vi "DS1104PlusDemo - 副本.vi"() -> ()   [LabVIEW 2018]
panel:
  out "错误输出":errorcluster
  in  "接口类型":u16(ring)=1 items=[""=0, "GPIB"=1, "VXI"=2, "GPIB-VXI"=3, "Serial"=4, "PXI"=5, "TCPIP"=6, "USB"=7, "FireWire"=9]
  in  "SINGLE Trigger":bool
  in  "RUN/STOP":bool
  in  "AUTO Set":bool
  in  "CLEAR Display":bool
  in  "Vertical Coupling":u16(ring) items=["AC", "DC", "Ground"]
  in  "Probe Attenuation":u16(ring) items=["1x"=1, "10x"=10]
  out "Single":bool caption="SINGLE"
  out "Normal":bool caption="NORMAL"
  out "Auto":bool caption="AUTO"
  in  "Trigger MODE":string(combo)
  in  "FORCE Trigger":bool
  in  "Trigger MENU":bool
  in  "Trigger LEVEL":dbl(ring)
  in  "Horizontal POSITION":ext format="%#_9g"
  in  "Horizontal MENU":bool
  in  "Horizaontal SCALE":ext(ring)=1e-09 items=["1u", "2u", "5u", "10u", "20u", "50u", "100u", "200u", "500u", "1m", "2m", "5m", "10m", "20m", "50m", "100m", "200m", "500m", "1", "2", "5", "10", "20", "50", "100", "200", "500", "1000"]
  in  "REF":bool
  in  "MATH":bool
  in  "Vertical SCALE":dbl(ring) items=["500u"=0.0005, "1m"=0.001, "2m"=0.002, "5m"=0.005, "10m"=0.01, "20m"=0.02, "50m"=0.05, "100m"=0.1, "200m"=0.2, "500m"=0.5, "1"=1.0, "2"=2.0, "5"=5.0, "10"=10.0, "20"=20.0, "50"=50.0, "100"=100.0]
  in  "Vertical POSITION":dbl min=-100.0 max=100.0 step=0.1 format="%#_4g"
  in  "CH4":bool
  in  "CH3":bool
  in  "CH2":bool
  in  "CH1":bool
  out "波形图":waveform(dbl)(graph)
  in  "VISA资源名称":refnum<visa-resource-name>
  # "VERTICAL"
  # "HORIZONTAL"
  # "TRIGGER"
  # "POSITION"
  # "POSITION"
  # "s"
  # "V"
  # "SCALE"
  # "SCALE"
  # "s/div"
  # "V/div"
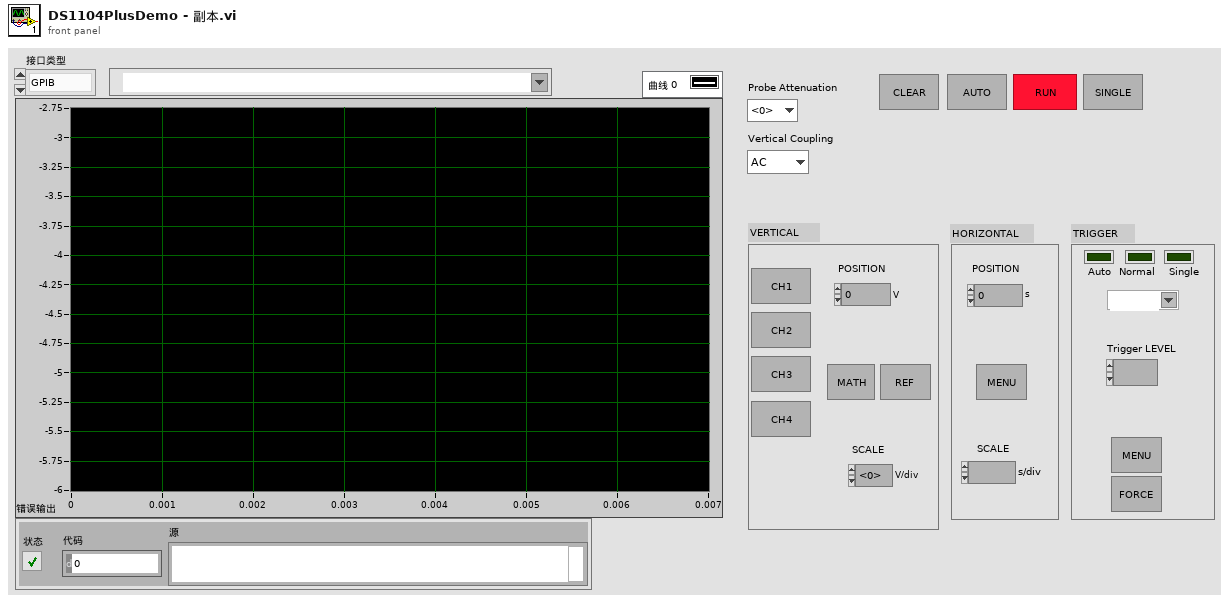
[diagram p1: front panel]
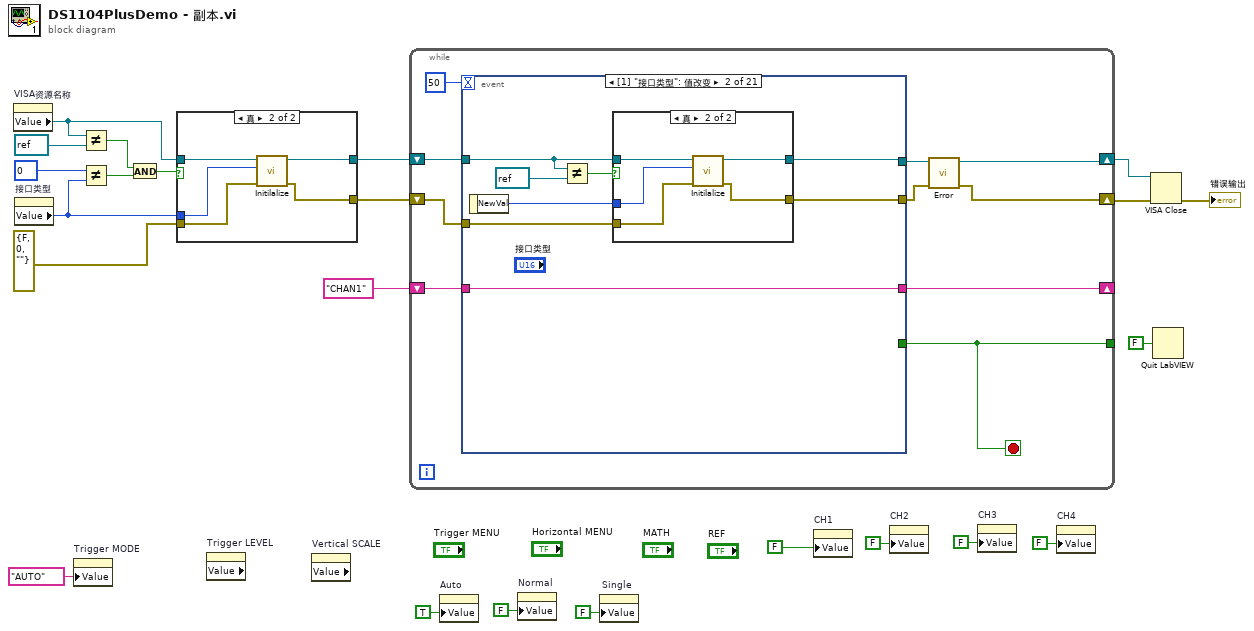
[diagram p0: block diagram]
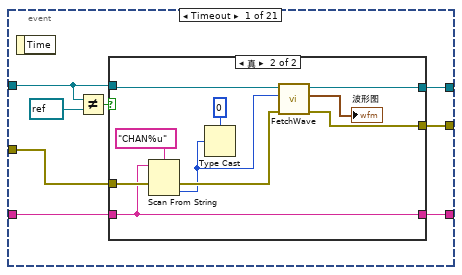
[diagram p3: hidden frame]
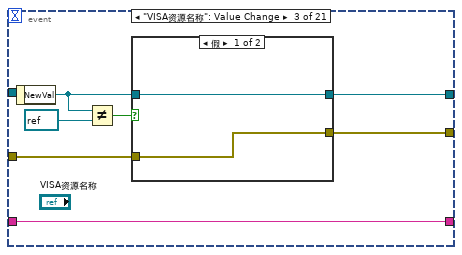
[diagram p6: hidden frame]
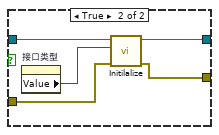
[diagram p7: hidden frame]
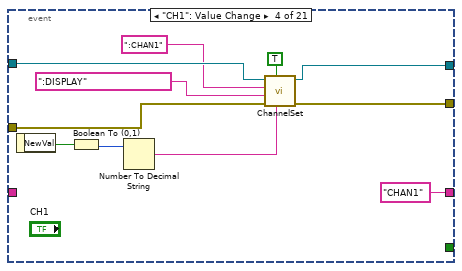
[diagram p8: hidden frame]
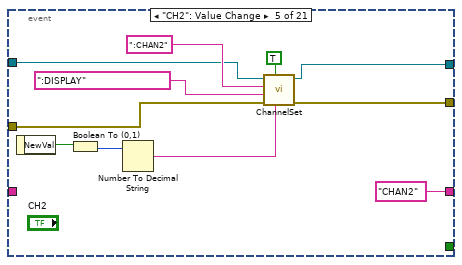
[diagram p9: hidden frame]
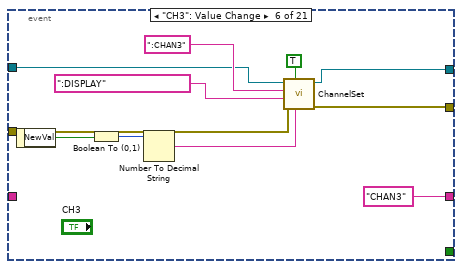
[diagram p10: hidden frame]
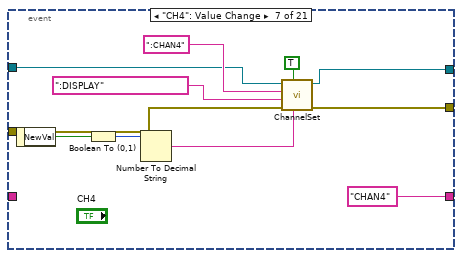
[diagram p11: hidden frame]
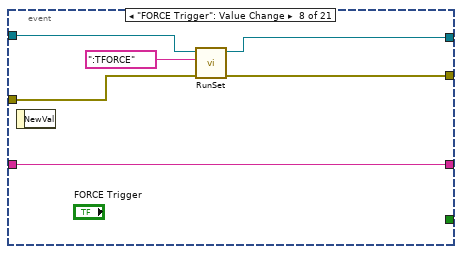
[diagram p12: hidden frame]
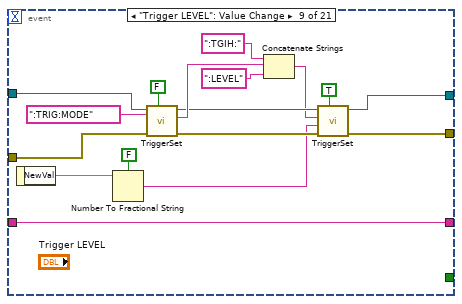
[diagram p13: hidden frame]
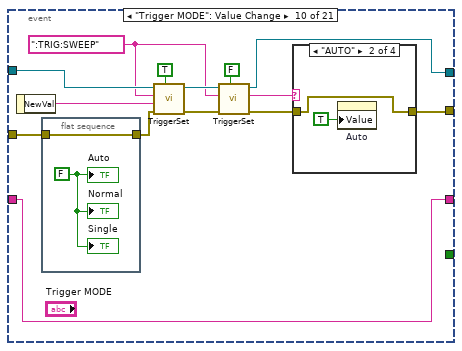
[diagram p14: hidden frame]
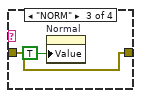
[diagram p16: hidden frame]
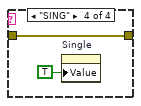
[diagram p17: hidden frame]
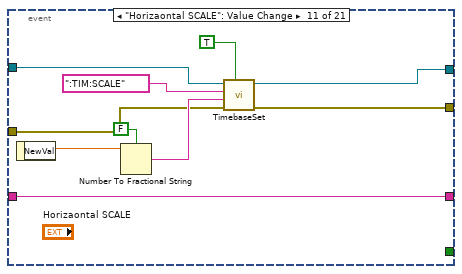
[diagram p18: hidden frame]
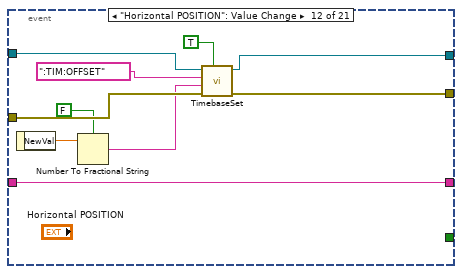
[diagram p19: hidden frame]
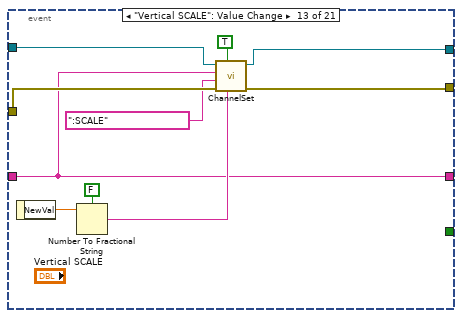
[diagram p20: hidden frame]
diagram:
  w12 = u16 0 items=[""=0, "GPIB"=1, "VXI"=2, "GPIB-VXI"=3, "Serial"=4, "PXI"=5, "TCPIP"=6, "USB"=7, "FireWire"=9] ("接口类型")
  n1 = property on="VISA资源名称" class="VISAName"() -> ("Value"=w13:refnum<visa-resource-name>)  [unwired: 2 in, 2 out]
  n2 = property on="接口类型" class="Ring (严格)"() -> ("Value"=w11:u16)  [unwired: 2 in, 2 out]
  n3 = property on="Trigger MODE" class="CmbBox"("Value"="AUTO" ("Trigger MODE")) -> ()  [unwired: 2 in, 2 out]
  n4 = Not Equal?(x=w13, y=refnum<visa-resource-name> refnum ("VISA引用句柄输出")) -> (x != y?=w16:bool)
  n5 = Not Equal?(x=w12, y=w11) -> (x != y?=w15:bool)
  n6 = And(x=w16, y=w15) -> (x .and. y?=w17:bool)
  n7 = case shown="真" w17 {
    tunnel: w13 -> [w25 w30]
    tunnel: errorcluster {"status"=FALSE, "code"=0, "source"=""} ("错误常量") -> [w24 w29]
    tunnel: w11 -> [_ w28]
    tunnel: [w24 w27] -> w9
    tunnel: [w25 w26] -> w10
    frame False {
    }
    frame True {
      n8 = call "Initilalize.vi"("错误输入（无错误）"=w29, "接口类型"=w28, "VISA资源名称"=w30) -> ("错误输出"=w27:errorcluster, "VISA资源名称输出"=w26:refnum<visa-resource-name>)  [unwired: 7 in]
    }
  }
  n9 = property on="Trigger LEVEL" class="Ring (严格)" props=["Value"]() -> ()  [unwired: 2 in, 3 out]
  n10 = property on="Vertical SCALE" class="Ring (严格)" props=["Value"]() -> ()  [unwired: 2 in, 3 out]
  n11 = while {
    shift-right: [w32] -> w8
    shift-left: w10 -> [w39]
    shift-right: [w33] -> w7
    shift-left: w9 -> [w38]
    shift-right: [w36] -> _
    shift-left: "CHAN1" ("通道选择") -> [w37]
    tunnel: [w31] -> _
    stop <- w31 stop-if-true
    n12 = event shown="[1] \"接口类型\": 值改变" {
      selector: _ -> [_ _ _ _ _ _ _ _ _ _ _ _ _ _ _ _ _ _ _ _ _]
      dyn-events: _ -> [_ _ _ _ _ _ _ _ _ _ _ _ _ _ _ _ _ _ _ _ _]
      timeout: 50 -> [_ _ _ _ _ _ _ _ _ _ _ _ _ _ _ _ _ _ _ _ _]
      tunnel: w39 -> [w42 w66 _ w101 w106 w119 w130 w138 w156 w171 w190 w199 w210 w218 w230 w236 w243 w249 w259 w264 w270]
      tunnel: w38 -> [w47 w65 w79 w100 w105 w118 w129 w139 w155 w159 w184 w200 w209 w217 w228 w239 w242 w250 w258 w265 w269]
      tunnel: [w46 w62 w78 w93 w104 w117 w128 w135 w141 w160 w183 w194 w204 w213 w227 w237 w241 w248 w257 w262 w267] -> w35
      tunnel: [w45 w63 w77 w92 w103 w116 w127 w137 w142 w161 w182 w193 w202 w212 w226 w238 w240 w247 w256 w261 w268] -> w34
      tunnel: w37 -> [w48 w69 w83 _ _ _ _ w140 w157 w170 w181 w192 w205 w211 w224 w235 w245 w251 w260 w266 w272]
      tunnel: [w41 w69 w83 "CHAN1" ("通道选择") "CHAN2" ("通道选择") "CHAN3" ("通道选择") "CHAN4" ("通道选择") w140 w157 w170 w181 w192 w205 w211 w224 w235 w245 w251 w260 w266 w271] -> w36
      tunnel: [_ _ _ _ _ _ _ _ _ _ _ _ _ _ _ _ _ _ _ _ w273] -> w31
      event Timeout {
        n13 = event-data() -> ()  [unwired: 1 in, 1 out]
        n14 = Not Equal?(x=w42, y=refnum<visa-resource-name> refnum) -> (x != y?=w44:bool)
        n15 = case shown="真" w44 {
          tunnel: w48 -> [w49 w54]
          tunnel: w47 -> [w50 w60]
          tunnel: [w51 w58] -> w46
          tunnel: [w50 w57] -> w45
          tunnel: w42 -> [w51 w55]
          tunnel: [w49 w54] -> w41
          frame False {
          }
          frame True {
            n16 = Scan From String(format string="CHAN%u" ("格式字符串"), input string=w54, error in=w60) -> (error out=w59:errorcluster, output 1=w52:u32)  [unwired: 2 in, 2 out]
            n17 = Type Cast(type=u16 0, x=w52) -> ()  [unwired: 1 out]
            n18 = call "FetchWave.vi"("error in (no error)"=w59, "通道"=w52, "VISA资源名称"=w55) -> ("error out"=w57:errorcluster, "波形图"=→"波形图":waveform(dbl), "VISA资源名称 2"=w58:refnum<visa-resource-name>)  [unwired: 6 in]
          }
        }
      }
      event "接口类型": Value Change {
        n19 = event-data() -> ("NewVal"=w64:u16)  [unwired: 1 in]
        n20 = Not Equal?(x=w66, y=refnum<visa-resource-name> refnum ("VISA引用句柄输出")) -> (x != y?=w67:bool)
        n21 = case shown="真" w67 {
          tunnel: w66 -> [w71 w76]
          tunnel: w65 -> [w70 w75]
          tunnel: w64 -> [_ w74]
          tunnel: [w70 w73] -> w63
          tunnel: [w71 w72] -> w62
          frame False {
          }
          frame True {
            n22 = call "Initilalize.vi"("错误输入（无错误）"=w75, "接口类型"=w74, "VISA资源名称"=w76) -> ("错误输出"=w73:errorcluster, "VISA资源名称输出"=w72:refnum<visa-resource-name>)  [unwired: 7 in]
          }
        }
      }
      event "VISA资源名称": Value Change {
        n23 = event-data() -> ("NewVal"=w80:refnum<visa-resource-name>)  [unwired: 1 in]
        n24 = Not Equal?(x=w80, y=refnum<visa-resource-name> refnum ("VISA引用句柄输出")) -> (x != y?=w81:bool)
        n25 = case shown="假" w81 {
          tunnel: w80 -> [w85 w90]
          tunnel: w79 -> [w84 w88]
          tunnel: [w85 w87] -> w78
          tunnel: [w84 w86] -> w77
          frame False {
          }
          frame True {
            n26 = property on="接口类型" class="Ring (严格)"() -> ("Value"=w89:u16)  [unwired: 2 in, 2 out]
            n27 = call "Initilalize.vi"("错误输入（无错误）"=w88, "接口类型"=w89, "VISA资源名称"=w90) -> ("错误输出"=w86:errorcluster, "VISA资源名称输出"=w87:refnum<visa-resource-name>)  [unwired: 7 in]
          }
        }
      }
      event "CH1": Value Change {
        n28 = event-data() -> ("NewVal"=w96:bool)  [unwired: 1 in]
        n29 = Boolean To (0,1)(Boolean=w96) -> (0, 1=w95:i16)
        n30 = Number To Decimal String(number=w95) -> (decimal integer string=w94:string)  [unwired: 1 in]
        n31 = call "ChannelSet.vi"("设置参数"=w94, "参数查询(0)/设置(1)"=TRUE, "error in (no error)"=w100, "CHANNLE命令子系统"=":DISPLAY", "通道选择"=":CHAN1", "VISA资源名称"=w101) -> ("error out"=w92:errorcluster, "VISA资源名称 2"=w93:refnum<visa-resource-name>)  [unwired: 2 in, 2 out]
      }
      event "CH2": Value Change {
        n32 = event-data() -> ("NewVal"=w102:bool)  [unwired: 1 in]
        n33 = Boolean To (0,1)(Boolean=w102) -> (0, 1=w110:i16)
        n34 = Number To Decimal String(number=w110) -> (decimal integer string=w109:string)  [unwired: 1 in]
        n35 = call "ChannelSet.vi"("设置参数"=w109, "参数查询(0)/设置(1)"=TRUE, "error in (no error)"=w105, "CHANNLE命令子系统"=":DISPLAY", "通道选择"=":CHAN2", "VISA资源名称"=w106) -> ("error out"=w103:errorcluster, "VISA资源名称 2"=w104:refnum<visa-resource-name>)  [unwired: 2 in, 2 out]
      }
      event "CH3": Value Change {
        n36 = event-data() -> ("NewVal"=w114:bool)  [unwired: 1 in]
        n37 = Boolean To (0,1)(Boolean=w114) -> (0, 1=w113:i16)
        n38 = Number To Decimal String(number=w113) -> (decimal integer string=w121:string)  [unwired: 1 in]
        n39 = call "ChannelSet.vi"("设置参数"=w121, "参数查询(0)/设置(1)"=TRUE, "error in (no error)"=w118, "CHANNLE命令子系统"=":DISPLAY", "通道选择"=":CHAN3", "VISA资源名称"=w119) -> ("error out"=w116:errorcluster, "VISA资源名称 2"=w117:refnum<visa-resource-name>)  [unwired: 2 in, 2 out]
      }
      event "CH4": Value Change {
        n40 = event-data() -> ("NewVal"=w125:bool)  [unwired: 1 in]
        n41 = Boolean To (0,1)(Boolean=w125) -> (0, 1=w124:i16)
        n42 = Number To Decimal String(number=w124) -> (decimal integer string=w132:string)  [unwired: 1 in]
        n43 = call "ChannelSet.vi"("设置参数"=w132, "参数查询(0)/设置(1)"=TRUE, "error in (no error)"=w129, "CHANNLE命令子系统"=":DISPLAY", "通道选择"=":CHAN4", "VISA资源名称"=w130) -> ("error out"=w127:errorcluster, "VISA资源名称 2"=w128:refnum<visa-resource-name>)  [unwired: 2 in, 2 out]
      }
      event "FORCE Trigger": Value Change {
        n44 = event-data() -> ()  [unwired: 1 in, 1 out]
        n45 = call "RunSet.vi"("error in (no error)"=w139, "TIMEBASE命令子系统"=":TFORCE", "VISA资源名称"=w138) -> ("error out"=w137:errorcluster, "VISA资源名称 2"=w135:refnum<visa-resource-name>)  [unwired: 7 in]
      }
      event "Trigger LEVEL": Value Change {
        n46 = event-data() -> ("NewVal"=w145:dbl)  [unwired: 1 in]
        n47 = Number To Fractional String(use system decimal point (T)=FALSE ("使用系统小数点(T)"), number=w145) -> (F-format string=w143:string)  [unwired: 2 in]
        n48 = call "TriggerSet.vi"("参数查询(0)/设置(1)"=FALSE, "error in (no error)"=w155, "TRIGGER命令子系统"=":TRIG:MODE", "VISA资源名称"=w156) -> ("error out"=w148:errorcluster, "查询返回"=w152:string, "VISA资源名称 2"=w149:refnum<visa-resource-name>)  [unwired: 4 in, 1 out]
        n49 = Concatenate Strings(":TGIH:" ("字符串"), w152, ":LEVEL" ("字符串")) -> (w147:string)
        n50 = call "TriggerSet.vi"("参数查询(0)/设置(1)"=TRUE, "error in (no error)"=w148, "设置参数"=w143, "TRIGGER命令子系统"=w147, "VISA资源名称"=w149) -> ("error out"=w142:errorcluster, "VISA资源名称 2"=w141:refnum<visa-resource-name>)  [unwired: 3 in, 2 out]
      }
      event "Trigger MODE": Value Change {
        w164 = ":TRIG:SWEEP" ("TRIGGER命令子系统")
        n51 = event-data() -> ("NewVal"=w168:string)  [unwired: 1 in]
        n52 = flat-sequence {
          tunnel: w159 -> [w173]
          tunnel: [w173] -> w158
          frame #0 {
            w172 = FALSE
            "Auto" <- w172
            "Normal" <- w172
            "Single" <- w172
          }
        }
        n53 = call "TriggerSet.vi"("参数查询(0)/设置(1)"=TRUE, "error in (no error)"=w158, "设置参数"=w168, "TRIGGER命令子系统"=w164, "VISA资源名称"=w171) -> ("error out"=w165:errorcluster, "VISA资源名称 2"=w167:refnum<visa-resource-name>)  [unwired: 3 in, 2 out]
        n54 = call "TriggerSet.vi"("参数查询(0)/设置(1)"=FALSE, "error in (no error)"=w165, "TRIGGER命令子系统"=w164, "VISA资源名称"=w167) -> ("error out"=w162:errorcluster, "查询返回"=w163:string, "VISA资源名称 2"=w160:refnum<visa-resource-name>)  [unwired: 4 in, 1 out]
        n55 = case shown="\"AUTO\"" w163 {
          tunnel: [w174 w175 w177 w179] -> w161
          tunnel: w162 -> [w174 w175 w177 w179]
          frame Default {
          }
          frame "AUTO" {
            n56 = property on="Auto" class="Bool (严格)"("Value"=TRUE ("Auto")) -> ()  [unwired: 2 in, 2 out]
          }
          frame "NORM" {
            n57 = property on="Normal" class="Bool (严格)"("Value"=TRUE ("Normal")) -> ()  [unwired: 2 in, 2 out]
          }
          frame "SING" {
            n58 = property on="Single" class="Bool (严格)"("Value"=TRUE ("Single")) -> ()  [unwired: 2 in, 2 out]
          }
        }
      }
      event "Horizaontal SCALE": Value Change {
        n59 = event-data() -> ("NewVal"=w186:ext)  [unwired: 1 in]
        n60 = Number To Fractional String(use system decimal point (T)=FALSE ("使用系统小数点(T)"), number=w186) -> (F-format string=w185:string)  [unwired: 2 in]
        n61 = call "TimebaseSet.vi"("参数查询(0)/设置(1)"=TRUE, "error in (no error)"=w184, "设置参数"=w185, "TIMEBASE命令子系统"=":TIM:SCALE", "VISA资源名称"=w190) -> ("error out"=w182:errorcluster, "VISA资源名称 2"=w183:refnum<visa-resource-name>)  [unwired: 3 in, 2 out]
      }
      event "Horizontal POSITION": Value Change {
        n62 = event-data() -> ("NewVal"=w191:ext)  [unwired: 1 in]
        n63 = Number To Fractional String(use system decimal point (T)=FALSE ("使用系统小数点(T)"), number=w191) -> (F-format string=w195:string)  [unwired: 2 in]
        n64 = call "TimebaseSet.vi"("参数查询(0)/设置(1)"=TRUE, "error in (no error)"=w200, "设置参数"=w195, "TIMEBASE命令子系统"=":TIM:OFFSET", "VISA资源名称"=w199) -> ("error out"=w193:errorcluster, "VISA资源名称 2"=w194:refnum<visa-resource-name>)  [unwired: 3 in, 2 out]
      }
      event "Vertical SCALE": Value Change {
        n65 = event-data() -> ("NewVal"=w201:dbl)  [unwired: 1 in]
        n66 = Number To Fractional String(use system decimal point (T)=FALSE ("使用系统小数点(T)"), number=w201) -> (F-format string=w207:string)  [unwired: 2 in]
        n67 = call "ChannelSet.vi"("设置参数"=w207, "参数查询(0)/设置(1)"=TRUE, "error in (no error)"=w209, "CHANNLE命令子系统"=":SCALE", "通道选择"=w205, "VISA资源名称"=w210) -> ("error out"=w202:errorcluster, "VISA资源名称 2"=w204:refnum<visa-resource-name>)  [unwired: 2 in, 2 out]
      }
      event "Vertical POSITION": Value Change {
        n68 = event-data() -> ("NewVal"=w216:dbl)  [unwired: 1 in]
        n69 = Number To Fractional String(use system decimal point (T)=FALSE ("使用系统小数点(T)"), number=w216) -> (F-format string=w214:string)  [unwired: 2 in]
        n70 = call "ChannelSet.vi"("设置参数"=w214, "参数查询(0)/设置(1)"=TRUE, "error in (no error)"=w217, "CHANNLE命令子系统"=":OFFSET", "通道选择"=w211, "VISA资源名称"=w218) -> ("error out"=w212:errorcluster, "VISA资源名称 2"=w213:refnum<visa-resource-name>)  [unwired: 2 in, 2 out]
      }
      event "Vertical Coupling": Value Change {
        n71 = event-data() -> ("NewVal"=w223:u16)  [unwired: 1 in]
        n72 = Pick Line(multi-line string="AC\nDC\nGND" ("多行字符串"), line index=w223) -> (output string=w221:string)  [unwired: 1 in]
        n73 = call "ChannelSet.vi"("设置参数"=w221, "参数查询(0)/设置(1)"=TRUE, "error in (no error)"=w228, "CHANNLE命令子系统"=":COUPLING", "通道选择"=w224, "VISA资源名称"=w230) -> ("error out"=w226:errorcluster, "VISA资源名称 2"=w227:refnum<visa-resource-name>)  [unwired: 2 in, 2 out]
      }
      event "Probe Attenuation": Value Change {
        # "设置指定模拟通道的探头衰减比"
        n74 = event-data() -> ("NewVal"=w233:u16)  [unwired: 1 in]
        n75 = Number To Fractional String(use system decimal point (T)=FALSE ("使用系统小数点(T)"), number=w233) -> (F-format string=w231:string)  [unwired: 2 in]
        n76 = call "ChannelSet.vi"("设置参数"=w231, "error in (no error)"=w239, "CHANNLE命令子系统"=":PROBE", "通道选择"=w235, "VISA资源名称"=w236) -> ("error out"=w238:errorcluster, "VISA资源名称 2"=w237:refnum<visa-resource-name>)  [unwired: 3 in, 2 out]
      }
      event "CLEAR Display": Value Change {
        n77 = event-data() -> ()  [unwired: 1 in, 1 out]
        n78 = call "RunSet.vi"("error in (no error)"=w242, "TIMEBASE命令子系统"=":CLEAR", "VISA资源名称"=w243) -> ("error out"=w240:errorcluster, "VISA资源名称 2"=w241:refnum<visa-resource-name>)  [unwired: 7 in]
      }
      event "AUTO Set": Value Change {
        n79 = event-data() -> ()  [unwired: 1 in, 1 out]
        n80 = call "RunSet.vi"("error in (no error)"=w250, "TIMEBASE命令子系统"=":AUTOSCALE", "VISA资源名称"=w249) -> ("error out"=w247:errorcluster, "VISA资源名称 2"=w248:refnum<visa-resource-name>)  [unwired: 7 in]
      }
      event "RUN/STOP": Value Change {
        n81 = event-data() -> ("NewVal"=w255:bool)  [unwired: 1 in]
        n82 = Select(t=":RUN" ("TIMEBASE命令子系统"), s=w255, f=":STOP" ("TIMEBASE命令子系统")) -> (s? t:f=w254:string)
        n83 = call "RunSet.vi"("error in (no error)"=w258, "TIMEBASE命令子系统"=w254, "VISA资源名称"=w259) -> ("error out"=w256:errorcluster, "VISA资源名称 2"=w257:refnum<visa-resource-name>)  [unwired: 7 in]
      }
      event "SINGLE Trigger": Value Change {
        n84 = event-data() -> ()  [unwired: 1 in, 1 out]
        n85 = call "RunSet.vi"("error in (no error)"=w265, "TIMEBASE命令子系统"=":SINGLE", "VISA资源名称"=w264) -> ("error out"=w261:errorcluster, "VISA资源名称 2"=w262:refnum<visa-resource-name>)  [unwired: 7 in]
      }
      event Menu Selection (User) {
        n86 = event-data() -> ("ItemTag"=w274:string)  [unwired: 1 in]
        n87 = case shown="\"退出\"" w274 {
          tunnel: [_ w280 _] -> w273
          tunnel: [w275 w281 w296] -> w271
          tunnel: w272 -> [w275 w282 w296]
          tunnel: w270 -> [w277 w284 w298]
          tunnel: w269 -> [w276 w283 w297]
          tunnel: [w276 w279 w297] -> w268
          tunnel: [w277 w278 w298] -> w267
          frame Default {
          }
          frame "退出" {
            n88 = Two Button Dialog(message="是否真的要退出程序？" ("消息")) -> (T button?=w285:bool)  [unwired: 2 in]
            n89 = case shown="假" w285 {
              selector: w285 -> [w289 w292]
              tunnel: w284 -> [w287 w295]
              tunnel: w283 -> [w288 w294]
              tunnel: [w290 w293] -> w281
              tunnel: w282 -> [w290 w293]
              tunnel: [w289 w292] -> w280
              tunnel: [w288 w291] -> w279
              tunnel: [w287 _] -> w278
              frame False {
              }
              frame True {
                n90 = call "Close.vi"("error in (no error)"=w294, "VISA资源名称"=w295) -> ("错误输出"=w291:errorcluster)  [unwired: 9 in]
              }
            }
          }
          frame "关于" {
          }
        }
      }
    }
    n91 = call "Error.vi"("error in (no error)"=w34, "VISA资源名称"=w35) -> ("错误输出"=w33:errorcluster, "VISA引用句柄输出"=w32:refnum<visa-resource-name>)  [unwired: 6 in, 2 out]
  }
  n92 = property on="Auto" class="Bool (严格)"("Value"=TRUE ("Auto")) -> ()  [unwired: 2 in, 2 out]
  n93 = property on="Normal" class="Bool (严格)"("Value"=FALSE ("Normal")) -> ()  [unwired: 2 in, 2 out]
  n94 = property on="Single" class="Bool (严格)"("Value"=FALSE ("Single")) -> ()  [unwired: 2 in, 2 out]
  n95 = property on="CH1" class="Bool (严格)"("Value"=FALSE ("CH1")) -> ()  [unwired: 2 in, 2 out]
  n96 = property on="CH2" class="Bool (严格)"("Value"=FALSE ("CH2")) -> ()  [unwired: 2 in, 2 out]
  n97 = property on="CH3" class="Bool (严格)"("Value"=FALSE ("CH3")) -> ()  [unwired: 2 in, 2 out]
  n98 = property on="CH4" class="Bool (严格)"("Value"=FALSE ("CH4")) -> ()  [unwired: 2 in, 2 out]
  n99 = VISA Close(VISA resource name=w8, error in (no error)=w7) -> (error out=→"错误输出":errorcluster)
  n100 = Quit LabVIEW(quit? (T)=FALSE ("退出？(T)")) -> ()
